vi "Choose selector.vi"(6 "wait for reply (T)":bool=TRUE, 8 "error in":errorcluster, 10 "Selector":i32, 11 "Module ID":i32=-1) -> (0 "error out":errorcluster, 1 "timed out?":bool, 3 "ID":dbl)   [LabVIEW 2020, in "TCP Client.lvlib"]
doc: "Choose the selector and change thing on client vi\n_____\nCreated using DQMH Event Scripter 6.0.0.122."
uses:
  TCP Client.lvlib
  Choose selector Argument--cluster.ctl
  Choose selector (Reply Payload)--cluster.ctl
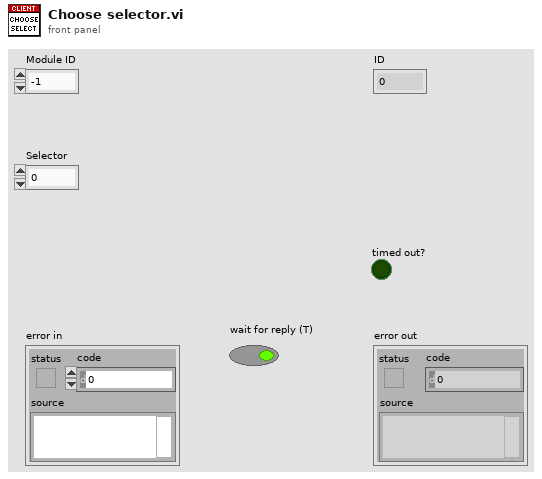
[diagram p1: front panel]
types:
  T1 = typedef "TCP Client.lvlib/Choose selector Argument--cluster.ctl" = cluster{"Module ID":i32, "Selector":i32, "Wait Notifier":refnum<notifier>, "wait for reply":bool}
  T2 = typedef "TCP Client.lvlib/Request Events--cluster.ctl" = cluster{"Stop Module":refnum<user-event>, "Show Panel":refnum<user-event>, "Hide Panel":refnum<user-event>, "Show Diagram":refnum<user-event>, "Get Module Execution Status":refnum<user-event>, "Connect To TCP Server":refnum<user-event>, "Choose selector":refnum<user-event>}
  T3 = typedef "TCP Client.lvlib/Choose selector (Reply Payload)--cluster.ctl" = cluster{"ID":dbl, "Choose selector_error":errorcluster}
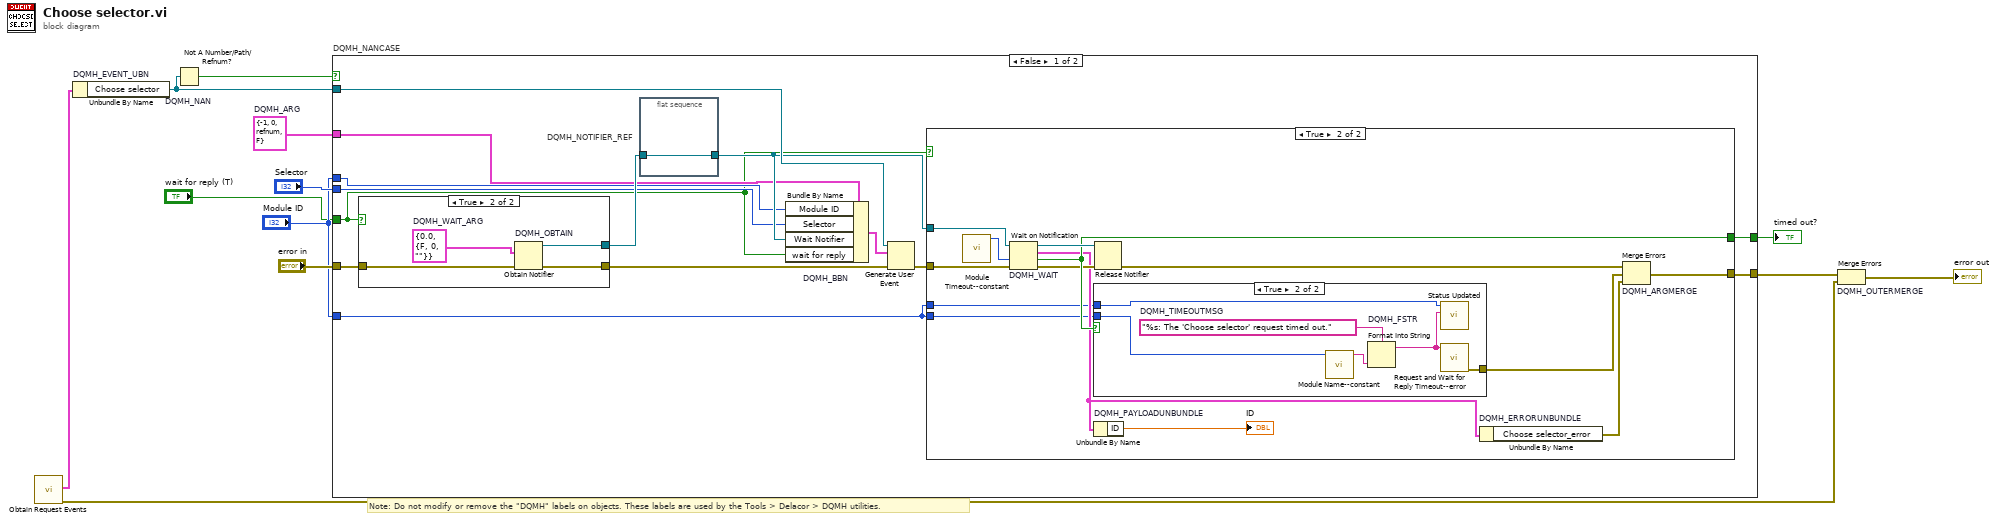
[diagram p0: block diagram]
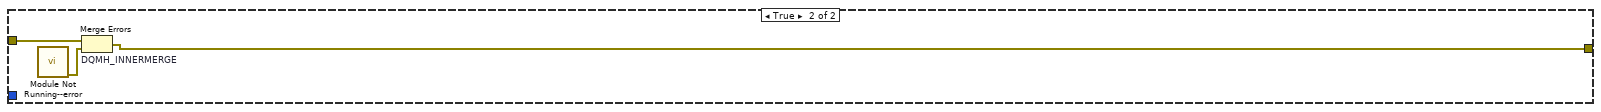
[diagram p5: hidden frame]
diagram:
  w6 = T1 {"Module ID"=-1, "Selector"=0, "Wait Notifier"=refnum, "wait for reply"=FALSE}  # DQMH_ARG
  # "Note: Do not modify or remove the \"DQMH\" labels on objects. These labels are used by the Tools > Delacor > DQMH utilities."
  n1 = call "Obtain Request Events.vi"() -> ("error out"=w2:errorcluster, "TCP Client Request Events"=w1:T2)  [unwired: 10 in]
  n2 = Unbundle By Name "DQMH_EVENT_UBN"(w1) -> ("Choose selector"=w10:refnum<user-event>)
  n3 = Not A Number/Path/Refnum? "DQMH_NAN"(number/path/refnum=w10) -> (NaN/Path/Refnum?=w9:bool)
  n4 = case "DQMH_NANCASE" shown="False" w9 {
    tunnel: "error in" -> [w26 w56]
    tunnel: w10 -> [w24 _]
    tunnel: [w21 w55] -> w7
    tunnel: [w22 _] -> w8
    tunnel: w6 -> [w17 _]
    tunnel: "Module ID" -> [w16 _]
    tunnel: "Selector" -> [w15 _]
    tunnel: "Module ID" -> [w14 _]
    tunnel: "wait for reply (T)" -> [w13 _]
    frame False {
      n5 = case shown="True" w13 {
        tunnel: w26 -> [w49 w53]
        tunnel: [w49 w52] -> w23
        tunnel: [_ w50] -> w19
        frame False {
        }
        frame True {
          w51 = T3 {"ID"=0.0, "Choose selector_error"={"status"=FALSE, "code"=0, "source"=""}}  # DQMH_WAIT_ARG
          n6 = Obtain Notifier "DQMH_OBTAIN"(notification data type=w51, error in (no error)=w53) -> (notifier out=w50:refnum<notifier>, error out=w52:errorcluster)  [unwired: 2 in, 1 out]
        }
      }
      n7 = flat-sequence "DQMH_NOTIFIER_REF" {
        tunnel: w19 -> [w27]
        tunnel: [w27] -> w18
        frame #0 {
        }
      }
      n8 = Bundle By Name "DQMH_BBN"(cluster=w17, "Module ID"=w16, "Selector"=w15, "Wait Notifier"=w18, "wait for reply"=w13) -> (w20:T1)
      n9 = Generate User Event(user event=w24, event data cluster=w20, error in=w23) -> (error out=w25:errorcluster)  [unwired: 1 in, 1 out]
      n10 = case shown="True" w13 {
        tunnel: w25 -> [w28 w42]
        tunnel: w18 -> [_ w41]
        tunnel: [_ w39] -> w22
        tunnel: [w28 w38] -> w21
        tunnel: w14 -> [_ w30]
        tunnel: w14 -> [_ w29]
        frame False {
        }
        frame True {
          n11 = call "Module Timeout--constant.vi"() -> ("Module Timeout"=w32:i32)  [unwired: 11 in]
          n12 = Wait on Notification "DQMH_WAIT"(notifier=w41, timeout in ms (-1)=w32, error in (no error)=w42) -> (notifier out=w40:refnum<notifier>, notification=w33:T3, timed out?=w39:bool, error out=w37:errorcluster)  [unwired: 1 in]
          n13 = case shown="True" w39 {
            tunnel: [_ w46] -> w34
            tunnel: w30 -> [_ w44]
            tunnel: w29 -> [_ w43]
            frame False {
            }
            frame True {
              w48 = "%s: The 'Choose selector' request timed out."  # DQMH_TIMEOUTMSG
              n14 = call "Module Name--constant.vi"("Module ID"=w43) -> ("Module Name"=w45:string)  [unwired: 10 in]
              n15 = Format Into String "DQMH_FSTR"(format string=w48, w45) -> (resulting string=w47:string)  [unwired: 2 in, 1 out]
              n16 = call "Status Updated.vi"("Status"=w47, "Module ID"=w44) -> ()  [unwired: 9 in, 1 out]
              n17 = call "Request and Wait for Reply Timeout--error.vi"("Error Message"=w47) -> ("error out"=w46:errorcluster)  [unwired: 10 in]
            }
          }
          n18 = Unbundle By Name "DQMH_PAYLOADUNBUNDLE"(w33) -> ("ID"=→"ID":dbl)
          n19 = Release Notifier(notifier=w40, error in (no error)=w37) -> (error out=w36:errorcluster)  [unwired: 1 in, 2 out]
          n20 = Unbundle By Name "DQMH_ERRORUNBUNDLE"(w33) -> ("Choose selector_error"=w35:errorcluster)
          n21 = Merge Errors "DQMH_ARGMERGE"(w36, w34, w35) -> (w38:errorcluster)
        }
      }
    }
    frame True {
      n22 = call "Module Not Running--error.vi"() -> ("error out"=w54:errorcluster)  [unwired: 11 in]
      n23 = Merge Errors "DQMH_INNERMERGE"(w56, w54) -> (w55:errorcluster)
    }
  }
  "timed out?" <- w8
  n24 = Merge Errors "DQMH_OUTERMERGE"(w7, w2) -> (→"error out":errorcluster)
